vi "test_connection.vi"(5 "読み取り前待機 (500 ms)":i16=500, 7 "文字送信間隔 (500 ms)":i16, 8 "error in (no error)":errorcluster caption="エラー入力（エラーなし）", 9 "想定レスポンス":string, 10 "コマンド":string, 11 "VISAリソース名":refnum<visa-resource-name>) -> (0 "error out":errorcluster caption="エラー出力", 1 "レスポンス":string, 2 "一致？":bool, 3 "VISAリソース名 （出力）":refnum<visa-resource-name>)   [LabVIEW 2017]
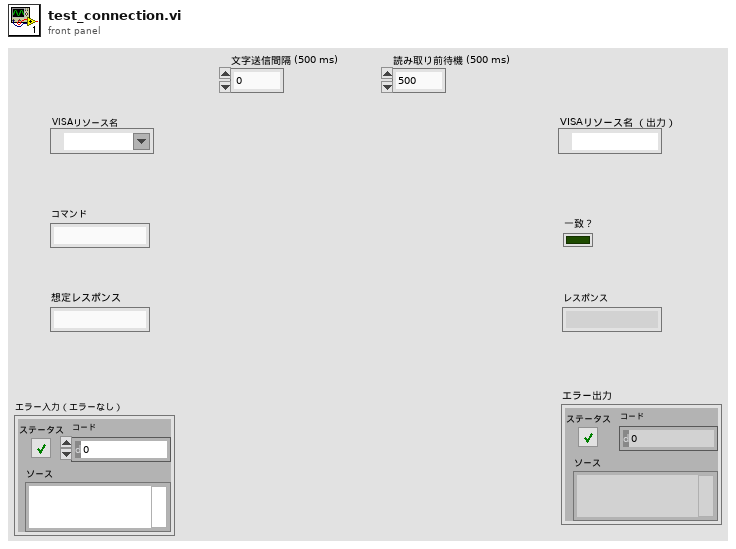
[diagram p1: front panel]
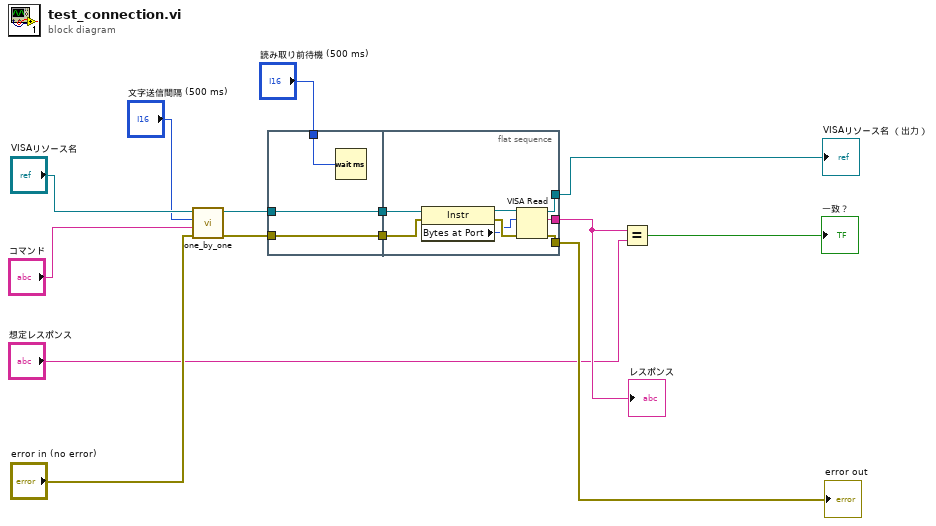
[diagram p0: block diagram]
diagram:
  n1 = call "one_by_one.vi"("error in (no error)"="error in (no error)", "入力文字"="コマンド", "待機 (200ms)"="文字送信間隔 (500 ms)", "VISAリソース名"="VISAリソース名") -> ("error out"=w10:errorcluster, "VISAリソース名出力"=w11:refnum<visa-resource-name>)  [unwired: 6 in]
  n2 = flat-sequence {
    tunnel: w10 -> [w16]
    tunnel: w11 -> [w17]
    tunnel: [w17] -> w4
    tunnel: [w16] -> w3
    tunnel: "読み取り前待機 (500 ms)" -> [w15]
    tunnel: [w20] -> w9
    tunnel: [w19] -> w8
    tunnel: [w18] -> w7
    tunnel: w4 -> [w25]
    tunnel: w3 -> [w24]
    frame #0 {
      n3 = Wait (ms)(milliseconds to wait=w15) -> ()  [unwired: 1 out]
    }
    frame #1 {
      n4 = property class="Instr"(reference=w25, error in=w24) -> (reference out=w23:refnum<visa-resource-name>, error out=w22:errorcluster, "Bytes at Port"=w21:u32)
      n5 = VISA Read(VISA resource name=w23, byte count=w21, error in (no error)=w22) -> (VISA resource name out=w19:refnum<visa-resource-name>, read buffer=w18:string, error out=w20:errorcluster)  [unwired: 1 out]
    }
  }
  n6 = Equal?(x=w7, y="想定レスポンス") -> (x = y?=→"一致？":bool)
  "VISAリソース名 （出力）" <- w8
  "レスポンス" <- w7
  "error out" <- w9
